vi "log analysis_gps.vi"() -> ()   [LabVIEW 2018] (continued)
 0 0\trobot status\t312.153988\t50.280852\t10.738100\t0.099388\t-2.098469\t148.636328\t0.292000\t0.008000\n\t\n15:31:20.4\tlog_raw\tgps_raw\t#DUALANTENNAHEADINGA,USB3,0,50.0,FINESTEERING,2107,282698.400,02000000,d426,15824;INSUFFICIENT_OBS,NONE,-1.000000000,0.000000000,0.000000000,0.0,0.000000000,0.000000000,\"631T\",17,3,3,3,04,00,20,00*5abb2bc4\n\tsystem status\tnormal 2 28.000000 0 0\trobot status\t312.043658\t50.366459\t10.734700\t0.055679\t-2.050793\t148.517573\t0.305000\t-0.006000\n\t\n15:31:20.9\tlog_raw\tgps_raw\t#DUALANTENNAHEADINGA,USB3,0,50.0,FINESTEERING,2107,282698.900,02000000,d426,15824;INSUFFICIENT_OBS,NONE,-1.000000000,0.000000000,0.000000000,0.0,0.000000000,0.000000000,\"631T\",17,3,3,3,04,00,20,00*e34415a1\n\tsystem status\tnormal 2 28.000000 0 0\trobot status\t311.931540\t50.455019\t10.731500\t0.131555\t-2.132212\t148.431701\t0.308000\t-0.012000\n\t\n15:31:21.4\tlog_raw\tgps_raw\t#DUALANTENNAHEADINGA,USB3,0,52.0,FINESTEERING,2107,282699.400,02000000,d426,15824;INSUFFICIENT_OBS,NONE,-1.000000000,0.000000000,0.000000000,0.0,0.000000000,0.000000000,\"631T\",17,3,3,3,04,00,20,00*ffea8255\n\tsystem status\tnormal 2 28.000000 0 0\trobot status\t311.824012\t50.539371\t10.729400\t0.149371\t-2.049793\t148.404291\t0.284000\t0.017000\n\t\n15:31:21.9\tlog_raw\tgps_raw\t#DUALANTENNAHEADINGA,USB3,0,52.0,FINESTEERING,2107,282699.900,02000000,d426,15824;INSUFFICIENT_OBS,NONE,-1.000000000,0.000000000,0.000000000,0.0,0.000000000,0.000000000,\"631T\",17,3,3,3,04,00,20,00*4615bc30\n\tsystem status\tnormal 2 28.000000 0 0\trobot status\t311.710632\t50.627656\t10.727600\t0.157188\t-2.016962\t148.331773\t0.246000\t0.060000\n\t\n15:31:22.4\tlog_raw\tgps_raw\t#DUALANTENNAHEADINGA,USB3,0,50.0,FINESTEERING,2107,282700.400,02000000,d426,15824;INSUFFICIENT_OBS,NONE,-1.000000000,0.000000000,0.000000000,0.0,0.000000000,0.000000000,\"631T\",12,3,3,3,04,00,20,00*82376373\n\tsystem status\tnormal 2 28.000000 0 0\trobot status\t311.597650\t50.714703\t10.723900\t0.029971\t-1.995727\t148.289238\t0.253000\t0.066000\n\t\n15:31:22.9\tlog_raw\tgps_raw\t#DUALANTENNAHEADINGA,USB3,0,50.0,FINESTEERING,2107,282700.900,02000000,d426,15824;INSUFFICIENT_OBS,NONE,-1.000000000,0.000000000,0.000000000,0.0,0.000000000,0.000000000,\"631T\",12,3,3,3,04,00,20,00*3bc85d16\n\tsystem status\tnormal 2 28.000000 0 0\trobot status\t311.486895\t50.801954\t10.721800\t-0.037655\t-1.925242\t148.274540\t0.292000\t0.015000\n\t\n15:31:23.4\tlog_raw\tgps_raw\t\tsystem status\tnormal 2 28.000000 0 0\trobot status\t311.374222\t50.890079\t10.718100\t-0.000984\t-1.833021\t148.262355\t0.287000\t0.023000\n\t\n15:31:23.9\tlog_raw\tgps_raw\t#INSPVAXA,USB3,0,51.0,FINESTEERING,2107,282701.950,02000000,471d,15824;INS_ALIGNMENT_COMPLETE,INS_RTKFIXED,37.37058966654,126.72434893958,10.7130,22.3000,0.1917,-0.1995,-0.0321,0.078081092,-1.836601738,301.669382711,0.4402,0.2934,0.5473,0.1136,0.0923,0.0770,0.0988,0.1035,4.8261,0f000001,0*8e2fcc51\n\tsystem status\tnormal 2 28.000000 0 0\trobot status\t311.249703\t50.988303\t10.713000\t0.078081\t-1.836602\t148.330617\t0.285000\t0.027000\n\t\n15:31:24.4\tlog_raw\tgps_raw\t\tsystem status\tnormal 2 28.000000 0 0\trobot status\t311.146061\t51.067657\t10.709700\t0.031833\t-1.930228\t148.322512\t0.245000\t0.078000\n\t\n15:31:24.9\tlog_raw\tgps_raw\t#DUALANTENNAHEADINGA,USB3,0,51.0,FINESTEERING,2107,282702.900,02000000,d426,15824;INSUFFICIENT_OBS,NONE,-1.000000000,0.000000000,0.000000000,0.0,0.000000000,0.000000000,\"631T\",15,3,3,3,04,00,20,00*ce02094b\n\tsystem status\tnormal 2 28.000000 0 0\trobot status\t311.034964\t51.152900\t10.708200\t-0.104424\t-1.731232\t148.345818\t0.298000\t0.001000\n\t\n15:31:25.4\tlog_raw\tgps_raw\t#INSPVAXA,USB3,0,51.0,FINESTEERING,2107,282703.450,02000000,471d,15824;INS_ALIGNMENT_COMPLETE,INS_RTKFIXED,37.37059201506,126.72434506763,10.7048,22.3000,0.1803,-0.1856,-0.0247,-0.105787498,-1.952133227,301.410927421,0.4394,0.2932,0.5469,0.1134,0.0923,0.0770,0.0988,0.1035,4.8271,0f000001,0*f23aaa81\n\tsystem status\tnormal 2 28.000000 0 0\trobot status\t310.906732\t51.248965\t10.704800\t-0.105787\t-1.952133\t148.589073\t0.305000\t0.000000\n\t\n15:31:25.9\tlog_raw\tgps_raw\t#INSPVAXA,USB3,0,51.0,FINESTEERING,2107,282703.950,02000000,471d,15824;INS_ALIGNMENT_COMPLETE,INS_RTKFIXED,37.37059277883,126.72434379347,10.7003,22.3000,0.1861,-0.1882,-0.0190,-0.127062602,-1.998823020,301.296665228,0.4394,0.2932,0.5469,0.1134,0.0923,0.0770,0.0988,0.1035,4.8271,0f000001,0*9cb21e47\n\tsystem status\tnormal 2 28.000000 0 0\trobot status\t310.793869\t51.333736\t10.700300\t-0.127063\t-1.998823\t148.703335\t0.249000\t0.075000\n\t\n15:31:26.4\tlog_raw\tgps_raw\t#INSPVAXA,USB3,0,45.5,FINESTEERING,2107,282704.450,02000000,471d,15824;INS_ALIGNMENT_COMPLETE,INS_RTKFIXED,37.37059354994,126.72434248772,10.6964,22.3000,0.1805,-0.1784,-0.0168,-0.125494848,-2.044475931,301.198188226,0.4393,0.2932,0.5468,0.1133,0.0923,0.0770,0.0987,0.1035,4.8275,0f000001,0*dae1e343\n\tsystem status\tnormal 2 28.000000 0 0\trobot status\t310.678208\t51.419322\t10.696400\t-0.125495\t-2.044476\t148.801812\t0.213000\t0.134000\n\t\n15:31:26.9\tlog_raw\tgps_raw\t#INSPVAXA,USB3,0,45.5,FINESTEERING,2107,282704.950,02000000,471d,15824;INS_ALIGNMENT_COMPLETE,INS_RTKFIXED,37.37059432216,126.72434118765,10.6925,22.3000,0.1836,-0.2007,-0.0268,-0.089569807,-2.221768291,301.087967534,0.4393,0.2932,0.5468,0.1133,0.0923,0.0770,0.0987,0.1035,4.8275,0f000001,0*2b6d582c\n\tsystem status\tnormal 2 28.000000 0 0\trobot status\t310.563050\t51.505031\t10.692500\t-0.089570\t-2.221768\t148.912032\t0.380000\t-0.104000\n\t\n15:31:27.4\tlog_raw\tgps_raw\t#DUALANTENNAHEADINGA,USB3,0,48.5,FINESTEERING,2107,282705.400,02000000,d426,15824;INSUFFICIENT_OBS,NONE,-1.000000000,0.000000000,0.000000000,0.0,0.000000000,0.000000000,\"631T\",14,3,3,3,04,00,20,00*0e4305d5\n\tsystem status\tnormal 2 28.000000 0 0\trobot status\t310.457755\t51.581804\t10.690600\t-0.088960\t-2.322934\t149.087146\t0.281000\t0.054000\n\t\n15:31:27.9\tlog_raw\tgps_raw\t#DUALANTENNAHEADINGA,USB3,0,48.5,FINESTEERING,2107,282705.900,02000000,d426,15824;INSUFFICIENT_OBS,NONE,-1.000000000,0.000000000,0.000000000,0.0,0.000000000,0.000000000,\"631T\",14,3,3,3,04,00,20,00*b7bc3bb0\n\tsystem status\tnormal 2 28.000000 0 0\trobot status\t310.344036\t51.665268\t10.686900\t-0.166864\t-2.273746\t149.175508\t0.358000\t-0.090000\n\t\n15:31:28.4\tlog_raw\tgps_raw\t#INSPVAXA,USB3,0,47.5,FINESTEERING,2107,282706.450,02000000,471d,15824;INS_ALIGNMENT_COMPLETE,INS_RTKFIXED,37.37059659513,126.72433727332,10.6837,22.3000,0.1676,-0.1882,-0.0314,-0.220175283,-2.295370003,300.572862367,0.4389,0.2931,0.5466,0.1133,0.0923,0.0770,0.0987,0.1035,4.8288,0f000001,0*8941e111\n\tsystem status\tnormal 2 28.000000 0 0\trobot status\t310.216325\t51.757308\t10.683700\t-0.220175\t-2.295370\t149.427138\t0.408000\t-0.162000\n\t\n15:31:28.9\tlog_raw\tgps_raw\t#DUALANTENNAHEADINGA,USB3,0,47.5,FINESTEERING,2107,282706.900,02000000,d426,15824;INSUFFICIENT_OBS,NONE,-1.000000000,0.000000000,0.000000000,0.0,0.000000000,0.000000000,\"631T\",11,3,3,3,04,00,20,00*4d3525fe\n\tsystem status\tnormal 2 27.900000 0 0\trobot status\t310.112312\t51.833880\t10.680500\t-0.168095\t-2.252926\t149.604257\t0.230000\t0.108000\n\t\n15:31:29.4\tlog_raw\tgps_raw\t#DUALANTENNAHEADINGA,USB3,0,52.0,FINESTEERING,2107,282707.400,02000000,d426,15824;INSUFFICIENT_OBS,NONE,-1.000000000,0.000000000,0.000000000,0.0,0.000000000,0.000000000,\"631T\",12,3,3,3,04,00,20,00*90c7d675\n\tsystem status\tnormal 2 28.000000 0 0\trobot status\t309.996490\t51.918113\t10.675200\t-0.123460\t-2.235362\t149.665344\t0.252000\t0.067000\n\t\n15:31:29.9\tlog_raw\tgps_raw\t#DUALANTENNAHEADINGA,USB3,0,52.0,FINESTEERING,2107,282707.900,02000000,d426,15824;INSUFFICIENT_OBS,NONE,-1.000000000,0.000000000,0.000000000,0.0,0.000000000,0.000000000,\"631T\",13,3,3,3,04,00,20,00*feda6848\n\tsystem status\tnormal 2 28.000000 0 0\trobot status\t309.880275\t52.002841\t10.669600\t-0.113111\t-2.188610\t149.711376\t0.209000\t0.130000\n\t\n15:31:30.4\tlog_raw\tgps_raw\t\tsystem status\tnormal 2 28.000000 0 0\trobot status\t309.762447\t52.086881\t10.664900\t-0.178646\t-2.254111\t149.746130\t0.246000\t0.084000\n\t\n15:31:30.9\tlog_raw\tgps_raw\t#DUALANTENNAHEADINGA,USB3,0,52.0,FINESTEERING,2107,282708.900,02000000,d426,15824;INSUFFICIENT_OBS,NONE,-1.000000000,0.000000000,0.000000000,0.0,0.000000000,0.000000000,\"631T\",15,3,3,3,04,00,20,00*615d515f\n\tsystem status\tnormal 2 28.000000 0 0\trobot status\t309.648645\t52.169373\t10.661300\t-0.273289\t-2.073858\t149.727816\t0.285000\t0.023000\n\t\n15:31:31.4\tlog_raw\tgps_raw\t#INSPVAXA,USB3,0,46.5,FINESTEERING,2107,282709.450,02000000,471d,15824;INS_ALIGNMENT_COMPLETE,INS_RTKFIXED,37.37060113294,126.72432942720,10.6558,22.3000,0.1792,-0.2126,-0.0198,-0.200491468,-1.971404566,300.268575337,0.4402,0.2931,0.5474,0.1135,0.0922,0.0770,0.0986,0.1035,4.8320,0f000001,0*91b882c4\n\tsystem status\tnormal 2 28.000000 0 0\trobot status\t309.521328\t52.260961\t10.655800\t-0.200491\t-1.971405\t149.731425\t0.346000\t-0.083000\n\t\n15:31:31.9\tlog_raw\tgps_raw\t#DUALANTENNAHEADINGA,USB3,0,46.5,FINESTEERING,2107,282709.900,02000000,d426,15824;INSUFFICIENT_OBS,NONE,-1.000000000,0.000000000,0.000000000,0.0,0.000000000,0.000000000,\"631T\",13,3,3,3,04,00,20,00*5f9ec7af\n\tsystem status\tnormal 2 28.000000 0 0\trobot status\t309.415133\t52.337101\t10.650600\t-0.241944\t-2.086526\t149.693208\t0.247000\t0.069000\n\t\n15:31:32.4\tlog_raw\tgps_raw\t#INSPVAXA,USB3,0,46.5,FINESTEERING,2107,282710.450,02000000,471d,15824;INS_ALIGNMENT_COMPLETE,INS_RTKFIXED,37.37060265280,126.72432675986,10.6463,22.3000,0.1745,-0.2044,-0.0168,-0.207189444,-2.098625918,300.356289546,0.4398,0.2931,0.5473,0.1134,0.0922,0.0770,0.0986,0.1035,4.8333,0f000001,0*cf6a9f79\n\tsystem status\tnormal 2 28.000000 0 0\trobot status\t309.285060\t52.429651\t10.646300\t-0.207189\t-2.098626\t149.643710\t0.289000\t0.013000\n\t\n15:31:32.9\tlog_raw\tgps_raw\t\tsystem status\tnormal 2 28.000000 0 0\trobot status\t309.181496\t52.504239\t10.642200\t-0.284971\t-2.151834\t149.572308\t0.358000\t-0.091000\n\t\n15:31:33.4\tlog_raw\tgps_raw\t#INSPVAXA,USB3,0,47.5,FINESTEERING,2107,282711.450,02000000,471d,15824;INS_ALIGNMENT_COMPLETE,INS_RTKFIXED,37.37060415509,126.72432413204,10.6400,22.3000,0.1796,-0.1977,-0.0235,-0.256481556,-2.212753880,300.512449739,0.4392,0.2930,0.5470,0.1133,0.0922,0.0770,0.0986,0.1035,4.8345,0f000001,0*c0ba1218\n\tsystem status\tnormal 2 28.000000 0 0\trobot status\t309.052292\t52.596390\t10.640000\t-0.256482\t-2.212754\t149.487550\t0.283000\t0.024000\n\t\n15:31:33.9\tlog_raw\tgps_raw\t\tsystem status\tnormal 2 28.000000 0 0\trobot status\t308.945130\t52.673510\t10.636200\t-0.199507\t-2.034759\t149.380948\t0.302000\t-0.013000\n\t\n15:31:34.4\tlog_raw\tgps_raw\t#INSPVAXA,USB3,0,47.5,FINESTEERING,2107,282712.450,02000000,471d,15824;INS_ALIGNMENT_COMPLETE,INS_RTKFIXED,37.37060568585,126.72432146015,10.6310,22.3000,0.1690,-0.1966,-0.0239,-0.257627218,-1.930020339,300.742925306,0.4385,0.2930,0.5468,0.1132,0.0922,0.0770,0.0986,0.1035,4.8358,0f000001,0*254ba6dd\n\tsystem status\tnormal 2 28.000000 0 0\trobot status\t308.815620\t52.766290\t10.631000\t-0.257627\t-1.930020\t149.257075\t0.289000\t0.004000\n\t\n15:31:34.9\tlog_raw\tgps_raw\t\tsystem status\tnormal 2 28.000000 0 0\trobot status\t308.713167\t52.840955\t10.626200\t-0.200836\t-1.765895\t149.148583\t0.301000\t-0.008000\n\t\n15:31:35.4\tlog_raw\tgps_raw\t#INSPVAXA,USB3,0,48.0,FINESTEERING,2107,282713.450,02000000,471d,15824;INS_ALIGNMENT_COMPLETE,INS_RTKFIXED,37.37060718735,126.72431885308,10.6223,22.3000,0.1755,-0.2010,-0.0238,-0.293375076,-1.794770522,300.954779767,0.4381,0.2930,0.5465,0.1133,0.0923,0.0770,0.0986,0.1035,4.8370,0f000001,0*2485d43a\n\tsystem status\tnormal 2 28.000000 0 0\trobot status\t308.584690\t52.932942\t10.622300\t-0.293375\t-1.794771\t149.045220\t0.299000\t-0.006000\n\t\n15:31:35.9\tlog_raw\tgps_raw\t#DUALANTENNAHEADINGA,USB3,0,48.0,FINESTEERING,2107,282713.900,02000000,d426,15824;INSUFFICIENT_OBS,NONE,-1.000000000,0.000000000,0.000000000,0.0,0.000000000,0.000000000,\"631T\",15,3,3,3,04,00,20,00*7de7f3c7\n\tsystem status\tnormal 2 28.000000 0 0\trobot status\t308.479465\t53.009824\t10.619200\t-0.302353\t-1.855203\t148.930937\t0.301000\t-0.010000\n\t\n15:31:36.4\tlog_raw\tgps_raw\t#INSPVAXA,USB3,0,50.5,FINESTEERING,2107,282714.450,02000000,471d,15824;INS_ALIGNMENT_COMPLETE,INS_RTKFIXED,37.37060872505,126.72431621182,10.6168,22.3000,0.1744,-0.1980,-0.0186,-0.254099040,-1.809317915,301.200596990,0.4382,0.2930,0.5463,0.1133,0.0922,0.0770,0.0986,0.1035,4.8379,0f000001,0*a4919b29\n\tsystem status\tnormal 2 28.000000 0 0\trobot status\t308.350731\t53.103611\t10.616800\t-0.254099\t-1.809318\t148.799403\t0.297000\t-0.004000\n\t\n15:31:36.9\tlog_raw\tgps_raw\t#INSPVAXA,USB3,0,50.5,FINESTEERING,2107,282714.950,02000000,471d,15824;INS_ALIGNMENT_COMPLETE,INS_RTKFIXED,37.37060951512,126.72431487294,10.6136,22.3000,0.1802,-0.2114,-0.0189,-0.186867307,-1.902236696,301.349579343,0.4382,0.2930,0.5463,0.1133,0.0922,0.0770,0.0986,0.1035,4.8379,0f000001,0*eb262157\n\tsystem status\tnormal 2 28.000000 0 0\trobot status\t308.232136\t53.191301\t10.613600\t-0.186867\t-1.902237\t148.650421\t0.300000\t-0.009000\n\t\n15:31:37.4\tlog_raw\tgps_raw\t#INSPVAXA,USB3,0,51.5,FINESTEERING,2107,282715.450,02000000,471d,15824;INS_ALIGNMENT_COMPLETE,INS_RTKFIXED,37.37061032466,126.72431346163,10.6103,22.3000,0.1848,-0.2311,-0.0198,-0.404081193,-1.989525185,301.491166671,0.4382,0.2930,0.5462,0.1132,0.0922,0.0770,0.0986,0.1035,4.8387,0f000001,0*760e8d75\n\tsystem status\tnormal 2 28.000000 0 0\trobot status\t308.107124\t53.281152\t10.610300\t-0.404081\t-1.989525\t148.508833\t0.310000\t-0.020000\n\t\n15:31:37.9\tlog_raw\tgps_raw\t\tsystem status\tnormal 2 28.000000 0 0\trobot status\t308.000122\t53.361998\t10.606800\t-0.274315\t-2.108873\t148.450181\t0.319000\t-0.047000\n\t\n15:31:38.4\tlog_raw\tgps_raw\t#INSPVAXA,USB3,0,45.5,FINESTEERING,2107,282716.450,02000000,471d,15824;INS_ALIGNMENT_COMPLETE,INS_RTKFIXED,37.37061184609,126.72431094127,10.6047,22.3000,0.1655,-0.1918,-0.0154,-0.319182162,-2.031673145,301.719710167,0.4383,0.2930,0.5462,0.1134,0.0922,0.0770,0.0985,0.1035,4.8397,0f000001,0*42f3853e\n\tsystem status\tnormal 2 28.000000 0 0\trobot status\t307.883875\t53.450016\t10.604700\t-0.319182\t-2.031673\t148.280290\t0.296000\t-0.006000\n\t\n15:31:38.9\tlog_raw\tgps_raw\t\tsystem status\tnormal 2 28.000000 0 0\trobot status\t307.778714\t53.528678\t10.602700\t-0.407200\t-2.039394\t148.201184\t0.297000\t-0.006000\n\t\n15:31:39.4\tlog_raw\tgps_raw\t#DUALANTENNAHEADINGA,USB3,0,47.5,FINESTEERING,2107,282717.400,02000000,d426,15824;INSUFFICIENT_OBS,NONE,-1.000000000,0.000000000,0.000000000,0.0,0.000000000,0.000000000,\"631T\",14,3,3,3,04,00,20,00*58fa208c\n\tsystem status\tnormal 2 28.000000 0 0\trobot status\t307.661116\t53.616622\t10.599900\t-0.484435\t-1.818123\t148.051820\t0.303000\t-0.005000\n\t\n15:31:39.9\tlog_raw\tgps_raw\t\tsystem status\tnormal 2 28.000000 0 0\trobot status\t307.544057\t53.706738\t10.596000\t-0.411925\t-1.602642\t147.906913\t0.307000\t-0.012000\n\t\n15:31:40.4\tlog_raw\tgps_raw\t#INSPVAXA,USB3,0,51.0,FINESTEERING,2107,282718.450,02000000,471d,15824;INS_ALIGNMENT_COMPLETE,INS_RTKFIXED,37.37061503275,126.72430567052,10.5915,22.3000,0.1670,-0.2003,-0.0156,-0.481720437,-1.537833901,302.225440084,0.4384,0.2930,0.5461,0.1133,0.0922,0.0770,0.0985,0.1035,4.8414,0f000001,0*c2621da1\n\tsystem status\tnormal 2 28.000000 0 0\trobot status\t307.417000\t53.803703\t10.591500\t-0.481720\t-1.537834\t147.774560\t0.294000\t0.004000\n\t\n15:31:40.9\tlog_raw\tgps_raw\t\tsystem status\tnormal 2 28.000000 0 0\trobot status\t307.319784\t53.880569\t10.587800\t-0.404063\t-1.530390\t147.667755\t0.297000\t-0.005000\n\t\n15:31:41.4\tlog_raw\tgps_raw\t#INSPVAXA,USB3,0,50.5,FINESTEERING,2107,282719.450,02000000,471d,15824;INS_ALIGNMENT_COMPLETE,INS_RTKFIXED,37.37061661000,126.72430311428,10.5856,22.3000,0.1775,-0.2289,-0.0225,-0.409943136,-1.702424996,302.531013260,0.4388,0.2931,0.5463,0.1134,0.0923,0.0770,0.0985,0.1035,4.8421,0f000001,0*cccf0b07\n\tsystem status\tnormal 2 28.000000 0 0\trobot status\t307.190573\t53.978762\t10.585600\t-0.409943\t-1.702425\t147.468987\t0.305000\t-0.011000\n\t\n15:31:41.9\tlog_raw\tgps_raw\t#INSPVAXA,USB3,0,50.5,FINESTEERING,2107,282719.950,02000000,471d,15824;INS_ALIGNMENT_COMPLETE,INS_RTKFIXED,37.37061741122,126.72430179575,10.5834,22.3000,0.1586,-0.2047,-0.0162,-0.368316866,-1.792689997,302.616582659,0.4388,0.2931,0.5463,0.1134,0.0923,0.0770,0.0985,0.1035,4.8421,0f000001,0*6a624589\n\tsystem status\tnormal 2 28.000000 0 0\trobot status\t307.073780\t54.067690\t10.583400\t-0.368317\t-1.792690\t147.383417\t0.295000\t0.003000\n\t\n15:31:42.4\tlog_raw\tgps_raw\t#INSPVAXA,USB3,0,52.5,FINESTEERING,2107,282720.450,02000000,471d,15824;INS_ALIGNMENT_COMPLETE,INS_RTKFIXED,37.37061822096,126.72430049242,10.5799,22.3000,0.1755,-0.2081,-0.0186,-0.303677811,-1.979848270,302.687255780,0.4391,0.2932,0.5464,0.1134,0.0923,0.0770,0.0985,0.1035,4.8427,0f000001,0*d8d179e3\n\tsystem status\tnormal 2 28.000000 0 0\trobot status\t306.958333\t54.157562\t10.579900\t-0.303678\t-1.979848\t147.312744\t0.352000\t-0.077000\n\t\n15:31:42.9\tlog_raw\tgps_raw\t#INSPVAXA,USB3,0,52.5,FINESTEERING,2107,282720.950,02000000,471d,15824;INS_ALIGNMENT_COMPLETE,INS_RTKFIXED,37.37061900063,126.72429922706,10.5769,22.3000,0.1781,-0.2246,-0.0135,-0.518744343,-1.838149425,302.751038564,0.4391,0.2932,0.5464,0.1134,0.0923,0.0770,0.0985,0.1035,4.8427,0f000001,0*0bb3f92c\n\tsystem status\tnormal 2 28.000000 0 0\trobot status\t306.846249\t54.244098\t10.576900\t-0.518744\t-1.838149\t147.248961\t0.369000\t-0.086000\n\t\n15:31:43.4\tlog_raw\tgps_raw\t#INSPVAXA,USB3,0,50.0,FINESTEERING,2107,282721.450,02000000,471d,15824;INS_ALIGNMENT_COMPLETE,INS_RTKFIXED,37.37061979310,126.72429796144,10.5749,22.3000,0.1738,-0.2158,-0.0193,-0.356246075,-1.735257546,302.750930181,0.4391,0.2932,0.5464,0.1133,0.0922,0.0770,0.0985,0.1035,4.8432,0f000001,0*0b05b843\n\tsystem status\tnormal 2 28.000000 0 0\trobot status\t306.734143\t54.332054\t10.574900\t-0.356246\t-1.735258\t147.249070\t0.261000\t0.059000\n\t\n15:31:43.9\tlog_raw\tgps_raw\t#INSPVAXA,USB3,0,50.0,FINESTEERING,2107,282721.950,02000000,471d,15824;INS_ALIGNMENT_COMPLETE,INS_RTKFIXED,37.37062058978,126.72429668610,10.5720,22.3000,0.1774,-0.2184,-0.0211,-0.236483678,-1.725198651,302.717948727,0.4391,0.2932,0.5464,0.1133,0.0922,0.0770,0.0985,0.1035,4.8432,0f000001,0*43a1a225\n\tsystem status\tnormal 2 28.000000 0 0\trobot status\t306.621175\t54.420477\t10.572000\t-0.236484\t-1.725199\t147.282051\t0.296000\t0.008000\n\t\n15:31:44.4\tlog_raw\tgps_raw\t#INSPVAXA,USB3,0,52.5,FINESTEERING,2107,282722.450,02000000,471d,15824;INS_ALIGNMENT_COMPLETE,INS_RTKFIXED,37.37062139294,126.72429536987,10.5676,22.3000,0.1685,-0.2034,-0.0272,-0.122026198,-1.692741983,302.685736194,0.4390,0.2932,0.5464,0.1133,0.0922,0.0770,0.0985,0.1034,4.8438,0f000001,0*76333eb5\n\tsystem status\tnormal 2 28.000000 0 0\trobot status\t306.504586\t54.509620\t10.567600\t-0.122026\t-1.692742\t147.314264\t0.390000\t-0.130000\n\t\n15:31:44.9\tlog_raw\tgps_raw\t#INSPVAXA,USB3,0,52.5,FINESTEERING,2107,282722.950,02000000,471d,15824;INS_ALIGNMENT_COMPLETE,INS_RTKFIXED,37.37062216038,126.72429408931,10.5632,22.3000,0.1618,-0.2145,-0.0280,-0.230140529,-1.688611156,302.634243103,0.4390,0.2932,0.5464,0.1133,0.0922,0.0770,0.0985,0.1034,4.8438,0f000001,0*93bbad2f\n\tsystem status\tnormal 2 28.000000 0 0\trobot status\t306.391156\t54.594798\t10.563200\t-0.230141\t-1.688611\t147.365757\t0.258000\t0.063000\n\t\n15:31:45.4\tlog_raw\tgps_raw\t\tsystem status\tnormal 2 28.000000 0 0\trobot status\t306.277993\t54.679518\t10.561200\t-0.219362\t-1.593746\t147.539828\t0.286000\t0.027000\n\t\n15:31:45.9\tlog_raw\tgps_raw\t#INSPVAXA,USB3,0,49.5,FINESTEERING,2107,282723.950,02000000,471d,15824;INS_ALIGNMENT_COMPLETE,INS_RTKFIXED,37.37062369834,126.72429151405,10.5583,22.3000,0.1641,-0.2086,-0.0359,-0.178637148,-1.711321137,302.326470730,0.4391,0.2932,0.5465,0.1133,0.0923,0.0770,0.0985,0.1034,4.8445,0f000001,0*3c6720b9\n\tsystem status\tnormal 2 28.000000 0 0\trobot status\t306.163043\t54.765496\t10.558300\t-0.178637\t-1.711321\t147.673529\t0.315000\t-0.015000\n\t\n15:31:46.4\tlog_raw\tgps_raw\t#INSPVAXA,USB3,0,45.0,FINESTEERING,2107,282724.450,02000000,471d,15824;INS_ALIGNMENT_COMPLETE,INS_RTKFIXED,37.37062445195,126.72429020244,10.5541,22.3000,0.1656,-0.2090,-0.0302,-0.201495719,-1.654592110,302.120912314,0.4391,0.2932,0.5466,0.1133,0.0923,0.0770,0.0985,0.1034,4.8452,0f000001,0*d09f31ec\n\tsystem status\tnormal 2 28.000000 0 0\trobot status\t306.046863\t54.849140\t10.554100\t-0.201496\t-1.654592\t147.879088\t0.275000\t0.036000\n\t\n15:31:46.9\tlog_raw\tgps_raw\t#INSPVAXA,USB3,0,45.0,FINESTEERING,2107,282724.950,02000000,471d,15824;INS_ALIGNMENT_COMPLETE,INS_RTKFIXED,37.37062519689,126.72428891232,10.5496,22.3000,0.1594,-0.2061,-0.0364,-0.113683805,-1.562683134,301.999815122,0.4391,0.2932,0.5466,0.1133,0.0923,0.0770,0.0985,0.1034,4.8452,0f000001,0*065bc9da\n\tsystem status\tnormal 2 27.900000 0 0\trobot status\t305.932586\t54.931821\t10.549600\t-0.113684\t-1.562683\t148.000185\t0.464000\t-0.244000\n\t\n15:31:47.4\tlog_raw\tgps_raw\t#INSPVAXA,USB3,0,52.5,FINESTEERING,2107,282725.450,02000000,471d,15824;INS_ALIGNMENT_COMPLETE,INS_RTKFIXED,37.37062594102,126.72428759328,10.5455,22.3000,0.1686,-0.2211,-0.0237,-0.147215314,-1.711523194,301.868011628,0.4387,0.2932,0.5466,0.1133,0.0923,0.0770,0.0985,0.1034,4.8461,0f000001,0*ee4f0d81\n\tsystem status\tnormal 2 27.900000 0 0\trobot status\t305.815748\t55.014412\t10.545500\t-0.147215\t-1.711523\t148.131988\t0.283000\t0.028000\n\t\n15:31:47.9\tlog_raw\tgps_raw\t#INSPVAXA,USB3,0,52.5,FINESTEERING,2107,282725.950,02000000,471d,15824;INS_ALIGNMENT_COMPLETE,INS_RTKFIXED,37.37062668932,126.72428627001,10.5411,22.3000,0.1745,-0.2284,-0.0369,-0.083032064,-1.696566260,301.720636014,0.4387,0.2932,0.5466,0.1133,0.0923,0.0770,0.0985,0.1034,4.8461,0f000001,0*1eb70b76\n\tsystem status\tnormal 2 28.000000 0 0\trobot status\t305.698535\t55.097466\t10.541100\t-0.083032\t-1.696566\t148.279364\t0.216000\t0.120000\n\t\n15:31:48.4\tlog_raw\tgps_raw\t\tsystem status\tnormal 2 28.000000 0 0\trobot status\t305.582363\t55.180138\t10.536700\t-0.107761\t-1.684703\t148.315471\t0.353000\t-0.082000\n\t\n15:31:48.9\tlog_raw\tgps_raw\t#INSPVAXA,USB3,0,51.5,FINESTEERING,2107,282726.950,02000000,471d,15824;INS_ALIGNMENT_COMPLETE,INS_RTKFIXED,37.37062817613,126.72428365004,10.5325,22.3000,0.1755,-0.2305,-0.0299,-0.122209734,-1.767911685,301.603525857,0.4391,0.2932,0.5469,0.1133,0.0923,0.0770,0.0985,0.1034,4.8469,0f000001,0*3fbc9b25\n\tsystem status\tnormal 2 28.000000 0 0\trobot status\t305.466462\t55.262488\t10.532500\t-0.122210\t-1.767912\t148.396474\t0.264000\t0.049000\n\t\n15:31:49.4\tlog_raw\tgps_raw\t#INSPVAXA,USB3,0,51.0,FINESTEERING,2107,282727.450,02000000,471d,15824;INS_ALIGNMENT_COMPLETE,INS_RTKFIXED,37.37062893743,126.72428230772,10.5272,22.3000,0.1765,-0.2181,-0.0244,-0.186365887,-1.943545299,301.556542913,0.4394,0.2932,0.5472,0.1133,0.0923,0.0770,0.0985,0.1034,4.8480,0f000001,0*c4ce36d4\n\tsystem status\tnormal 2 28.000000 0 0\trobot status\t305.347562\t55.346985\t10.527200\t-0.186366\t-1.943545\t148.443457\t0.220000\t0.099000\n\t\n15:31:49.9\tlog_raw\tgps_raw\t#INSPVAXA,USB3,0,51.0,FINESTEERING,2107,282727.950,02000000,471d,15824;INS_ALIGNMENT_COMPLETE,INS_RTKFIXED,37.37062969227,126.72428097983,10.5215,22.3000,0.1787,-0.2040,-0.0183,-0.254427310,-1.978392002,301.576926117,0.4394,0.2932,0.5472,0.1133,0.0923,0.0770,0.0985,0.1034,4.8480,0f000001,0*e99e732b\n\tsystem status\tnormal 2 28.000000 0 0\trobot status\t305.229940\t55.430764\t10.521500\t-0.254427\t-1.978392\t148.423074\t0.243000\t0.083000\n\t\n15:31:50.4\tlog_raw\tgps_raw\t\tsystem status\tnormal 2 28.000000 0 0\trobot status\t305.113678\t55.516327\t10.518400\t-0.141860\t-1.956111\t148.395592\t0.258000\t0.063000\n\t\n15:31:50.9\tlog_raw\tgps_raw\t#INSPVAXA,USB3,0,51.5,FINESTEERING,2107,282728.950,02000000,471d,15824;INS_ALIGNMENT_COMPLETE,INS_RTKFIXED,37.37063122299,126.72427838355,10.5148,22.3000,0.1885,-0.2208,-0.0203,-0.119828900,-1.930080778,301.638982245,0.4399,0.2933,0.5477,0.1134,0.0923,0.0770,0.0984,0.1034,4.8492,0f000001,0*2b605f5c\n\tsystem status\tnormal 2 28.000000 0 0\trobot status\t304.999965\t55.600659\t10.514800\t-0.119829\t-1.930081\t148.361018\t0.296000\t0.022000\n\t\n15:31:51.4\tlog_raw\tgps_raw\t\tsystem status\tnormal 2 28.000000 0 0\trobot status\t304.883247\t55.687933\t10.510500\t-0.194587\t-1.878840\t148.199095\t0.334000\t-0.058000\n\t\n15:31:51.9\tlog_raw\tgps_raw\t#INSPVAXA,USB3,0,52.5,FINESTEERING,2107,282729.950,02000000,471d,15824;INS_ALIGNMENT_COMPLETE,INS_RTKFIXED,37.37063278846,126.72427577866,10.5058,22.3000,0.1873,-0.2222,-0.0212,-0.280509981,-1.724312983,301.915248261,0.4403,0.2933,0.5480,0.1134,0.0923,0.0770,0.0984,0.1035,4.8506,0f000001,0*b7f0a5a5\n\tsystem status\tnormal 2 28.000000 0 0\trobot status\t304.769228\t55.774411\t10.505800\t-0.280510\t-1.724313\t148.084752\t0.308000\t-0.018000\n\t\n15:31:52.4\tlog_raw\tgps_raw\t#INSPVAXA,USB3,0,51.5,FINESTEERING,2107,282730.450,02000000,471d,15824;INS_ALIGNMENT_COMPLETE,INS_RTKFIXED,37.37063357878,126.72427449323,10.5033,22.3000,0.1727,-0.2057,-0.0242,-0.264377135,-1.835119150,302.025936707,0.4422,0.2933,0.5491,0.1137,0.0923,0.0771,0.0985,0.1035,4.8518,0f000001,0*7f6e5cf1\n\tsystem status\tnormal 2 28.000000 0 0\trobot status\t304.655367\t55.862128\t10.503300\t-0.264377\t-1.835119\t147.974063\t0.293000\t0.001000\n\t\n15:31:52.9\tlog_raw\tgps_raw\t\tsystem status\tnormal 2 28.000000 0 0\trobot status\t304.542702\t55.949278\t10.501200\t-0.319487\t-2.042561\t147.881198\t0.300000\t-0.001000\n\t\n15:31:53.4\tlog_raw\tgps_raw\t#INSPVAXA,USB3,0,49.0,FINESTEERING,2107,282731.450,02000000,471d,15824;INS_ALIGNMENT_COMPLETE,INS_RTKFIXED,37.37063518922,126.72427189807,10.4972,22.3000,0.1874,-0.2156,-0.0321,-0.243858308,-2.166120506,302.258331909,0.4432,0.2934,0.5498,0.1138,0.0924,0.0771,0.0985,0.1035,4.8531,0f000001,0*8b4646cd\n\tsystem status\tnormal 2 28.000000 0 0\trobot status\t304.425492\t56.040871\t10.497200\t-0.243858\t-2.166121\t147.741668\t0.304000\t-0.011000\n\t\n15:31:53.9\tlog_raw\tgps_raw\t#INSPVAXA,USB3,0,49.0,FINESTEERING,2107,282731.950,02000000,471d,15824;INS_ALIGNMENT_COMPLETE,INS_RTKFIXED,37.37063597309,126.72427066217,10.4933,22.3000,0.1763,-0.1976,-0.0267,-0.212826377,-2.311379439,302.361551522,0.4432,0.2934,0.5498,0.1138,0.0924,0.0771,0.0985,0.1035,4.8531,0f000001,0*776c7422\n\tsystem status\tnormal 2 28.000000 0 0\trobot status\t304.316018\t56.127872\t10.493300\t-0.212826\t-2.311379\t147.638448\t0.276000\t0.018000\n\t\n15:31:54.4\tlog_raw\tgps_raw\t\tsystem status\tnormal 2 28.000000 0 0\trobot status\t304.196736\t56.221869\t10.489400\t-0.166625\t-2.521388\t147.542465\t0.275000\t0.035000\n\t\n15:31:54.9\tlog_raw\tgps_raw\t\tsystem status\tnormal 2 28.000000 0 0\trobot status\t304.091091\t56.307582\t10.485600\t-0.278464\t-2.470936\t147.446319\t0.306000\t-0.011000\n\t\n15:31:55.4\tlog_raw\tgps_raw\t\tsystem status\tnormal 2 28.000000 0 0\trobot status\t303.974611\t56.401212\t10.481100\t-0.341795\t-2.420035\t147.324160\t0.279000\t0.029000\n\t\n15:31:55.9\tlog_raw\tgps_raw\t#INSPVAXA,USB3,0,48.5,FINESTEERING,2107,282733.950,02000000,471d,15824;INS_ALIGNMENT_COMPLETE,INS_RTKFIXED,37.37063924201,126.72426559710,10.4772,22.3000,0.2027,-0.2332,-0.0277,-0.317088293,-2.273099501,302.707061030,0.4435,0.2934,0.5506,0.1138,0.0925,0.0772,0.0985,0.1035,4.8550,0f000001,0*95b7724f\n\tsystem status\tnormal 2 28.000000 0 0\trobot status\t303.867363\t56.490688\t10.477200\t-0.317088\t-2.273100\t147.292939\t0.295000\t0.026000\n\t\n15:31:56.4\tlog_raw\tgps_raw\t#INSPVAXA,USB3,0,48.5,FINESTEERING,2107,282734.450,02000000,471d,15824;INS_ALIGNMENT_COMPLETE,INS_RTKFIXED,37.37064005686,126.72426435901,10.4738,22.3000,0.1910,-0.2119,-0.0289,-0.216766474,-2.387675538,302.660035367,0.4432,0.2934,0.5508,0.1138,0.0925,0.0772,0.0985,0.1036,4.8555,0f000001,0*b9d42d58\n\tsystem status\tnormal 2 28.000000 0 0\trobot status\t303.757695\t56.581128\t10.473800\t-0.216766\t-2.387676\t147.339965\t0.287000\t0.013000\n\t\n15:31:56.9\tlog_raw\tgps_raw\t\tsystem status\tnormal 2 28.000000 0 0\trobot status\t303.643754\t56.674024\t10.470100\t-0.208217\t-2.511260\t147.363019\t0.285000\t0.013000\n\t\n15:31:57.4\tlog_raw\tgps_raw\t\tsystem status\tnormal 2 28.000000 0 0\trobot status\t303.532403\t56.763863\t10.467100\t-0.191643\t-2.642967\t147.459456\t0.244000\t0.096000\n\t\n15:31:57.9\tlog_raw\tgps_raw\t\tsystem status\tnormal 2 28.000000 0 0\trobot status\t303.419632\t56.854171\t10.463200\t-0.219764\t-2.711653\t147.647524\t0.219000\t0.126000\n\t\n15:31:58.4\tlog_raw\tgps_raw\t\tsystem status\tnormal 2 27.900000 0 0\trobot status\t303.305800\t56.943297\t10.458900\t-0.230574\t-2.719547\t147.832322\t0.351000\t-0.083000\n\t\n15:31:58.9\tlog_raw\tgps_raw\t\tsystem status\tnormal 2 27.900000 0 0\trobot status\t303.194393\t57.029373\t10.453600\t-0.348612\t-2.556803\t148.049896\t0.220000\t0.117000\n\t\n15:31:59.4\tlog_raw\tgps_raw\t\tsystem status\tnormal 2 28.000000 0 0\trobot status\t303.084061\t57.114078\t10.450700\t-0.264868\t-2.244077\t148.382455\t0.234000\t0.093000\n\t\n15:31:59.9\tlog_raw\tgps_raw\t\tsystem status\tnormal 2 27.900000 0 0\trobot status\t302.970475\t57.199856\t10.449100\t-0.266418\t-2.230726\t148.666670\t0.314000\t-0.006000\n\t\n15:32:00.4\tlog_raw\tgps_raw\t\tsystem status\tnormal 2 27.900000 0 0\trobot status\t302.855402\t57.284802\t10.446300\t-0.346059\t-2.067029\t148.857680\t0.397000\t-0.151000\n\t\n15:32:00.9\tlog_raw\tgps_raw\t\tsystem status\tnormal 2 27.900000 0 0\trobot status\t302.741408\t57.369041\t10.442200\t-0.403669\t-1.863817\t149.004585\t0.213000\t0.132000\n\t\n15:32:01.4\tlog_raw\tgps_raw\t\tsystem status\tnormal 2 27.900000 0 0\trobot status\t302.625361\t57.453457\t10.439300\t-0.364718\t-1.887757\t149.172771\t0.208000\t0.147000\n\t\n15:32:01.9\tlog_raw\tgps_raw\t\tsystem status\tnormal 2 28.000000 0 0\trobot status\t302.509180\t57.538126\t10.435100\t-0.316403\t-2.082701\t149.255239\t0.361000\t-0.090000\n\t\n15:32:02.4\tlog_raw\tgps_raw\t\tsystem status\tnormal 2 28.000000 0 0\trobot status\t302.393503\t57.620189\t10.432400\t-0.428981\t-2.061326\t149.336466\t0.360000\t-0.088000\n\t\n15:32:02.9\tlog_raw\tgps_raw\t\tsystem status\tnormal 2 28.000000 0 0\trobot status\t302.278460\t57.702179\t10.430400\t-0.543285\t-2.118903\t149.421890\t0.279000\t0.025000\n\t\n15:32:03.4\tlog_raw\tgps_raw\t\tsystem status\tnormal 2 28.000000 0 0\trobot status\t302.160807\t57.785618\t10.427700\t-0.519066\t-2.351140\t149.467894\t0.290000\t0.014000\n\t\n15:32:03.9\tlog_raw\tgps_raw\t\tsystem status\tnormal 2 28.000000 0 0\trobot status\t302.045849\t57.868895\t10.424000\t-0.430859\t-2.396997\t149.427489\t0.317000\t-0.048000\n\t\n15:32:04.4\tlog_raw\tgps_raw\t\tsystem status\tnormal 2 28.000000 0 0\trobot status\t301.929806\t57.953133\t10.421300\t-0.470180\t-2.367430\t149.325446\t0.228000\t0.095000\n\t\n15:32:04.9\tlog_raw\tgps_raw\t\tsystem status\tnormal 2 28.000000 0 0\trobot status\t301.813660\t58.039707\t10.420000\t-0.410930\t-2.367914\t149.171409\t0.313000\t-0.020000\n\t\n15:32:05.4\tlog_raw\tgps_raw\t\tsystem status\tnormal 2 28.000000 0 0\trobot status\t301.697856\t58.124301\t10.417300\t-0.494168\t-2.536440\t149.071086\t0.299000\t0.000000\n\t\n15:32:05.9\tlog_raw\tgps_raw\t\tsystem status\tnormal 2 28.000000 0 0\trobot status\t301.572425\t58.215921\t10.412400\t-0.459715\t-2.588552\t149.036420\t0.237000\t0.088000\n\t\n15:32:06.4\tlog_raw\tgps_raw\t\tsystem status\tnormal 2 28.000000 0 0\trobot status\t301.467163\t58.293498\t10.409100\t-0.626344\t-2.620838\t148.864288\t0.308000\t-0.013000\n\t\n15:32:06.9\tlog_raw\tgps_raw\t\tsystem status\tnormal 2 28.000000 0 0\trobot status\t301.342433\t58.385784\t10.405600\t-0.523357\t-2.807271\t148.732795\t0.285000\t0.018000\n\t\n15:32:07.4\tlog_raw\tgps_raw\t#INSPVAXA,USB3,0,46.0,FINESTEERING,2107,282745.450,02000000,471d,15824;INS_ALIGNMENT_COMPLETE,INS_RTKFIXED,37.37065707294,126.72423583291,10.4038,22.3000,0.1644,-0.2205,-0.0248,-0.393666989,-2.802189375,301.368033402,0.4424,0.2935,0.5497,0.1137,0.0923,0.0771,0.0985,0.1035,4.8609,0f000001,0*4c364312\n\tsystem status\tnormal 2 28.000000 0 0\trobot status\t301.230899\t58.469742\t10.403800\t-0.393667\t-2.802189\t148.631967\t0.306000\t-0.017000\n\t\n15:32:07.9\tlog_raw\tgps_raw\t\tsystem status\tnormal 2 28.000000 0 0\trobot status\t301.103974\t58.562999\t10.400300\t-0.327028\t-2.854228\t148.608617\t0.221000\t0.114000\n\t\n15:32:08.4\tlog_raw\tgps_raw\t\tsystem status\tnormal 2 28.000000 0 0\trobot status\t300.995876\t58.643924\t10.398100\t-0.358783\t-2.745504\t148.469096\t0.302000\t-0.007000\n\t\n15:32:08.9\tlog_raw\tgps_raw\t\tsystem status\tnormal 2 28.000000 0 0\trobot status\t300.869890\t58.735880\t10.394200\t-0.425854\t-2.848587\t148.427920\t0.317000\t-0.028000\n\t\n15:32:09.4\tlog_raw\tgps_raw\t\tsystem status\tnormal 2 28.000000 0 0\trobot status\t300.760507\t58.817987\t10.391400\t-0.515558\t-2.878329\t148.336350\t0.267000\t0.045000\n\t\n15:32:09.9\tlog_raw\tgps_raw\t\tsystem status\tnormal 2 28.000000 0 0\trobot status\t300.649903\t58.902704\t10.389400\t-0.495948\t-2.703320\t148.222829\t0.300000\t-0.002000\n\t\n15:32:10.4\tlog_raw\tgps_raw\t\tsystem status\tnormal 2 28.000000 0 0\trobot status\t300.527225\t58.992917\t10.386100\t-0.652838\t-2.532503\t148.134728\t0.301000\t-0.006000\n\t\n15:32:10.9\tlog_raw\tgps_raw\t\tsystem status\tnormal 2 28.000000 0 0\trobot status\t300.417410\t59.077159\t10.383300\t-0.586380\t-2.410385\t148.023340\t0.258000\t0.062000\n\t\n15:32:11.4\tlog_raw\tgps_raw\t\tsystem status\tnormal 2 28.000000 0 0\trobot status\t300.302955\t59.164696\t10.379300\t-0.494965\t-2.323340\t147.885077\t0.304000\t-0.019000\n\t\n15:32:11.9\tlog_raw\tgps_raw\t\tsystem status\tnormal 2 28.000000 0 0\trobot status\t300.184974\t59.253752\t10.375000\t-0.609369\t-2.264935\t147.854232\t0.349000\t-0.078000\n\t\n15:32:12.4\tlog_raw\tgps_raw\t\tsystem status\tnormal 2 28.000000 0 0\trobot status\t300.068803\t59.341682\t10.370400\t-0.764369\t-2.625045\t147.679709\t0.307000\t-0.010000\n\t\n15:32:12.9\tlog_raw\tgps_raw\t\tsystem status\tnormal 2 28.000000 0 0\trobot status\t299.950578\t59.431592\t10.365200\t-0.739895\t-2.999679\t147.770368\t0.268000\t0.046000\n\t\n15:32:13.4\tlog_raw\tgps_raw\t\tsystem status\tnormal 2 28.000000 0 0\trobot status\t299.840165\t59.515710\t10.360900\t-0.675094\t-3.219075\t147.657260\t0.313000\t-0.011000\n\t\n15:32:13.9\tlog_raw\tgps_raw\t\tsystem status\tnormal 2 28.000000 0 0\trobot status\t299.719108\t59.606371\t10.356000\t-0.677024\t-3.573825\t147.598902\t0.277000\t0.036000\n\t\n15:32:14.4\tlog_raw\tgps_raw\t\tsystem status\tnormal 2 28.000000 0 0\trobot status\t299.602180\t59.692286\t10.351000\t-0.804178\t-3.532671\t147.517442\t0.304000\t-0.007000\n\t\n15:32:15.0\tlog_raw\tgps_raw\t\tsystem status\tnormal 2 28.000000 0 0\trobot status\t299.488910\t59.774562\t10.345300\t-1.145070\t-3.489461\t147.492768\t0.362000\t-0.098000\n\t\n15:32:15.5\tlog_raw\tgps_raw\t\tsystem status\tnormal 2 28.000000 0 0\trobot status\t299.369477\t59.862155\t10.337800\t-1.619685\t-3.454526\t147.465061\t0.262000\t0.049000\n\t\n15:32:16.0\tlog_raw\tgps_raw\t\tsystem status\tnormal 2 28.000000 0 0\trobot status\t299.256652\t59.948686\t10.331400\t-1.728304\t-3.382839\t147.428860\t0.302000\t0.001000\n\t\n15:32:16.5\tlog_raw\tgps_raw\t\tsystem status\tnormal 2 28.000000 0 0\trobot status\t299.144170\t60.035664\t10.325800\t-1.803553\t-3.351963\t147.466715\t0.255000\t0.069000\n\t\n15:32:17.0\tlog_raw\tgps_raw\t\tsystem status\tnormal 2 28.000000 0 0\trobot status\t299.030148\t60.123170\t10.320900\t-1.969028\t-3.203508\t147.448613\t0.301000\t-0.010000\n\t\n15:32:17.5\tlog_raw\tgps_raw\t\tsystem status\tnormal 2 28.000000 0 0\trobot status\t298.917163\t60.211028\t10.316400\t-2.103433\t-2.879673\t147.477019\t0.367000\t-0.086000\n\t\n15:32:18.0\tlog_raw\tgps_raw\t\tsystem status\tnormal 2 28.000000 0 0\trobot status\t298.807005\t60.297444\t10.312800\t-2.192038\t-2.552253\t147.501466\t0.325000\t-0.045000\n\t\n15:32:18.5\tlog_raw\tgps_raw\t\tsystem status\tnormal 2 28.000000 0 0\trobot status\t298.694267\t60.384960\t10.308600\t-2.275810\t-2.224480\t147.530342\t0.301000\t-0.007000\n\t\n15:32:19.0\tlog_raw\tgps_raw\t\tsystem status\tnormal 2 28.000000 0 0\trobot status\t298.581389\t60.474472\t10.304000\t-2.177401\t-2.111520\t147.626958\t0.256000\t0.066000\n\t\n15:32:19.5\tlog_raw\tgps_raw\t\tsystem status\tnormal 2 28.000000 0 0\trobot status\t298.466555\t60.563024\t10.299000\t-2.070453\t-2.265005\t147.634892\t0.261000\t0.063000\n\t\n15:32:20.0\tlog_raw\tgps_raw\t\tsystem status\tnormal 2 28.000000 0 0\trobot status\t298.353982\t60.650229\t10.294700\t-1.891583\t-2.295388\t147.725703\t0.226000\t0.085000\n\t\n15:32:20.5\tlog_raw\tgps_raw\t\tsystem status\tnormal 2 28.000000 0 0\trobot status\t298.237533\t60.740931\t10.290600\t-1.719454\t-2.537720\t147.855835\t0.227000\t0.089000\n\t\n15:32:21.0\tlog_raw\tgps_raw\t\tsystem status\tnormal 2 28.000000 0 0\trobot status\t298.121763\t60.830877\t10.285200\t-1.645270\t-2.648518\t147.950728\t0.402000\t-0.155000\n\t\n15:32:21.5\tlog_raw\tgps_raw\t\tsystem status\tnormal 2 28.000000 0 0\trobot status\t298.008019\t60.919262\t10.277800\t-1.564126\t-2.764192\t148.082054\t0.379000\t-0.129000\n\t\n15:32:22.0\tlog_raw\tgps_raw\t\tsystem status\tnormal 2 28.000000 0 0\trobot status\t297.895062\t61.007115\t10.270200\t-1.483299\t-2.682272\t148.156607\t0.332000\t-0.067000\n\t\n15:32:22.5\tlog_raw\tgps_raw\t\tsystem status\tnormal 2 28.000000 0 0\trobot status\t297.777506\t61.096541\t10.262200\t-1.394864\t-2.896060\t148.309912\t0.261000\t0.051000\n\t\n15:32:23.0\tlog_raw\tgps_raw\t\tsystem status\tnormal 2 28.000000 0 0\trobot status\t297.661636\t61.184249\t10.254300\t-1.412182\t-3.126366\t148.391590\t0.250000\t0.079000\n\t\n15:32:23.5\tlog_raw\tgps_raw\t\tsystem status\tnormal 2 28.000000 0 0\trobot status\t297.547960\t61.271484\t10.245100\t-1.334373\t-3.167686\t148.451303\t0.289000\t0.019000\n\t\n15:32:24.0\tlog_raw\tgps_raw\t\tsystem status\tnormal 2 28.000000 0 0\trobot status\t297.431186\t61.359581\t10.234700\t-1.330328\t-3.571292\t148.572456\t0.398000\t-0.155000\n\t\n15:32:24.5\tlog_raw\tgps_raw\t\tsystem status\tnormal 2 28.000000 0 0\trobot status\t297.310077\t61.446775\t10.223500\t-1.543736\t-4.227686\t148.631227\t0.222000\t0.109000\n\t\n15:32:25.0\tlog_raw\tgps_raw\t\tsystem status\tnormal 2 28.000000 0 0\trobot status\t297.193894\t61.529484\t10.211900\t-1.810619\t-4.621180\t148.643525\t0.360000\t-0.089000\n\t\n15:32:25.5\tlog_raw\tgps_raw\t\tsystem status\tnormal 2 28.000000 0 0\trobot status\t297.077659\t61.614249\t10.201200\t-1.813111\t-4.968623\t148.734432\t0.365000\t-0.100000\n\t\n15:32:26.0\tlog_raw\tgps_raw\t\tsystem status\tnormal 2 28.000000 0 0\trobot status\t296.959814\t61.700626\t10.189000\t-1.723971\t-5.255245\t148.717260\t0.358000\t-0.092000\n\t\n15:32:26.5\tlog_raw\tgps_raw\t\tsystem status\tnormal 2 28.000000 0 0\trobot status\t296.847255\t61.782301\t10.177300\t-1.730567\t-4.861590\t148.782254\t0.355000\t-0.088000\n\t\n15:32:27.0\tlog_raw\tgps_raw\t\tsystem status\tnormal 2 28.000000 0 0\trobot status\t296.739340\t61.860985\t10.167700\t-1.775299\t-4.185156\t148.761672\t0.238000\t0.094000\n\t\n15:32:27.5\tlog_raw\tgps_raw\t\tsystem status\tnormal 2 28.000000 0 0\trobot status\t296.626624\t61.944355\t10.157800\t-1.688239\t-3.803296\t148.734853\t0.268000\t0.036000\n\t\n15:32:28.0\tlog_raw\tgps_raw\t#INSPVAXA,USB3,0,50.5,FINESTEERING,2107,282766.000,02000000,471d,15824;INS_ALIGNMENT_COMPLETE,INS_RTKFIXED,37.37068918572,126.72418251405,10.1497,22.3000,0.1565,-0.2244,-0.0284,-1.470427926,-2.806836785,301.304662044,0.4416,0.2936,0.5519,0.1137,0.0923,0.0773,0.0984,0.1037,4.8731,0f000001,0*1edafe1a\n\tsystem status\tnormal 2 28.000000 0 0\trobot status\t296.508002\t62.033935\t10.149700\t-1.470428\t-2.806837\t148.695338\t0.286000\t0.036000\n\t\n15:32:28.5\tlog_raw\tgps_raw\t#INSPVAXA,USB3,0,48.0,FINESTEERING,2107,282766.500,
